vi "MeasureSinglePulse.vi"   [LabVIEW 2019]
uses:
  Global/Global Variables/global.vi
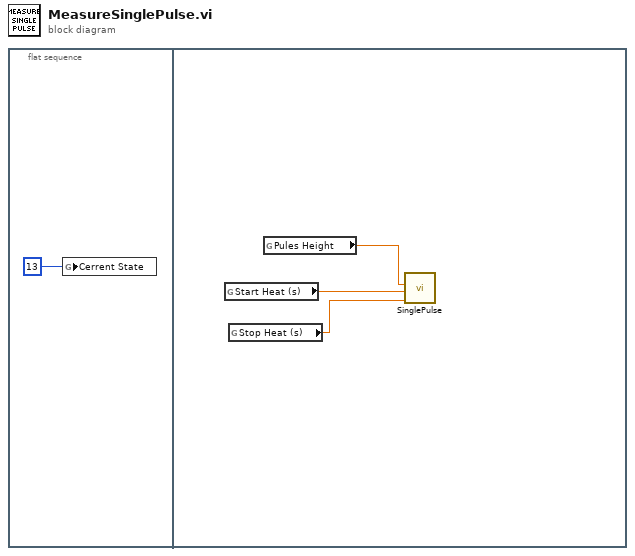
[diagram p0: block diagram]
diagram:
  n1 = flat-sequence {
    frame #0 {
      n2 = global write "global.vi" "Cerrent State"(13) -> ()
    }
    frame #1 {
      n3 = global read "global.vi" "Start Heat (s)"() -> (w3:dbl)
      n4 = global read "global.vi" "Stop Heat (s)"() -> (w2:dbl)
      n5 = global read "global.vi" "Pules Height"() -> (w4:dbl)
      n6 = call "SinglePulse.vi"("Stop heat (s)"=w2, "Start heat (s)"=w3, "Pulse Height (A) 2"=w4) -> ()  [unwired: 4 in, 5 out]
    }
  }
